vi "Memory Size Enum to Numeric.vi"(8 "error in (no error)":errorcluster, 11 "FPGA Memory Size":T1) -> (0 "error out":errorcluster, 3 "Numeric":i32)   [LabVIEW 2011, in "Engine Sim System Explorer.lvlib"]
uses:
  Engine Sim System Explorer.lvlib
  TypeDefs/FPGA Mem Size.ctl
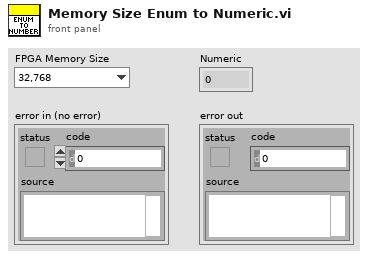
[diagram p1: front panel]
types:
  T1 = typedef "Engine Sim System Explorer.lvlib/FPGA Mem Size.ctl" = enum16{"32,768", "16,384", "8,192", "4,096", "2,048", "1024", "512", "256", "128"}
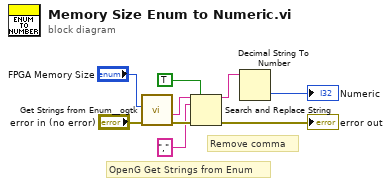
[diagram p0: block diagram]
diagram:
  # "Remove comma"
  # "OpenG Get Strings from Enum"
  n1 = call <userlib>:"Get Strings from Enum__ogtk.vi"("error in (no error)"="error in (no error)", "Enum"="FPGA Memory Size") -> ("error out"=w7:errorcluster, "String Value"=w4:string)  [unwired: 6 in, 2 out]
  n2 = Search and Replace String(replace all?=TRUE ("replace all? (F)"), input string=w4, search string=",", error in=w7) -> (result string=w3:string, error out=→"error out":errorcluster)  [unwired: 4 in, 2 out]
  n3 = Decimal String To Number(string=w3) -> (number=→"Numeric":i32)  [unwired: 2 in, 1 out]
